vi "SetLaserConfigLCDC501.vi"(2 "LASER CONFIGURATION":T1={"LD Range"=1, "Laser Control Mode"=0, "Laser Mod On/OFF"=1, "Laser Mod BW"=1} {"Laser Mod BW" items=["Low", "High"]; "Laser Mod On/OFF" items=["OFF", "ON"]; "Laser Control Mode" items=["CC", "CP"]; "LD Range" items=["250mA", "500mA"]}, 8 "error in (no error)":errorcluster, 11 "VISA resource name":refnum<visa-resource-name>) -> (0 "error out":errorcluster, 3 "VISA resource name out":refnum<visa-resource-name>)   [LabVIEW 2021]
panel:
  # "LD Currernt Range"
  # "Laser Control Mode"
  # "Laser Mod On/OFF"
  # "Laser Mod BW"
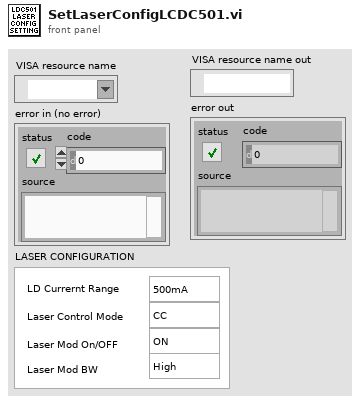
[diagram p1: front panel]
types:
  T1 = cluster{"LD Range":u16, "Laser Control Mode":u16, "Laser Mod On/OFF":u16, "Laser Mod BW":u16}
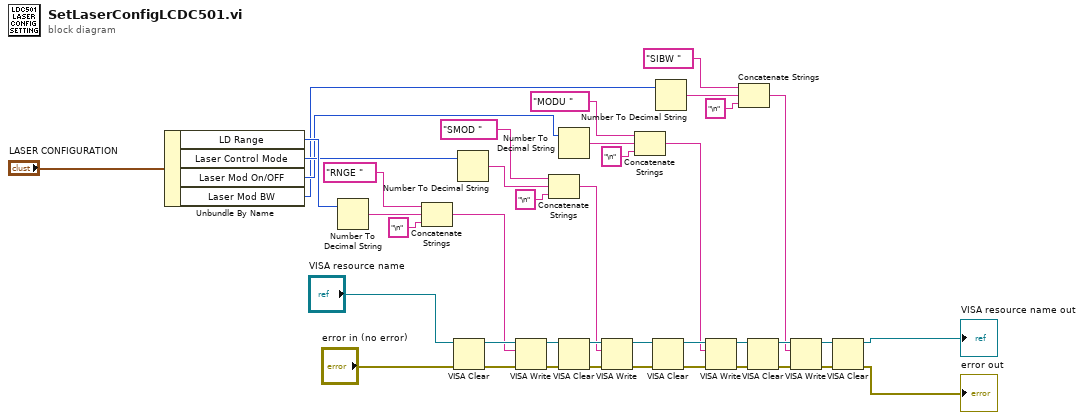
[diagram p0: block diagram]
diagram:
  n1 = Unbundle By Name("LASER CONFIGURATION") -> ("LD Range"=w6:u16, "Laser Control Mode"=w5:u16, "Laser Mod On/OFF"=w4:u16, "Laser Mod BW"=w3:u16)
  n2 = Number To Decimal String(number=w6) -> (decimal integer string=w31:string)  [unwired: 1 in]
  n3 = Concatenate Strings("RNGE " ("write buffer"), w31, "\n" ("string")) -> (w28:string)
  n4 = VISA Clear(VISA resource name="VISA resource name", error in (no error)="error in (no error)") -> (VISA resource name out=w40:refnum<visa-resource-name>, error out=w41:errorcluster)
  n5 = Number To Decimal String(number=w5) -> (decimal integer string=w26:string)  [unwired: 1 in]
  n6 = VISA Write(VISA resource name=w40, write buffer=w28, error in (no error)=w41) -> (VISA resource name out=w24:refnum<visa-resource-name>, error out=w23:errorcluster)  [unwired: 1 out]
  n7 = Concatenate Strings("SMOD " ("write buffer"), w26, "\n" ("string")) -> (w22:string)
  n8 = Number To Decimal String(number=w4) -> (decimal integer string=w17:string)  [unwired: 1 in]
  n9 = VISA Clear(VISA resource name=w24, error in (no error)=w23) -> (VISA resource name out=w38:refnum<visa-resource-name>, error out=w39:errorcluster)
  n10 = VISA Write(VISA resource name=w38, write buffer=w22, error in (no error)=w39) -> (VISA resource name out=w21:refnum<visa-resource-name>, error out=w20:errorcluster)  [unwired: 1 out]
  n11 = Concatenate Strings("MODU " ("write buffer"), w17, "\n" ("string")) -> (w16:string)
  n12 = VISA Clear(VISA resource name=w21, error in (no error)=w20) -> (VISA resource name out=w36:refnum<visa-resource-name>, error out=w37:errorcluster)
  n13 = Number To Decimal String(number=w3) -> (decimal integer string=w12:string)  [unwired: 1 in]
  n14 = VISA Write(VISA resource name=w36, write buffer=w16, error in (no error)=w37) -> (VISA resource name out=w15:refnum<visa-resource-name>, error out=w14:errorcluster)  [unwired: 1 out]
  n15 = Concatenate Strings("SIBW " ("write buffer"), w12, "\n" ("string")) -> (w10:string)
  n16 = VISA Clear(VISA resource name=w15, error in (no error)=w14) -> (VISA resource name out=w34:refnum<visa-resource-name>, error out=w35:errorcluster)
  n17 = VISA Write(VISA resource name=w34, write buffer=w10, error in (no error)=w35) -> (VISA resource name out=w9:refnum<visa-resource-name>, error out=w8:errorcluster)  [unwired: 1 out]
  n18 = VISA Clear(VISA resource name=w9, error in (no error)=w8) -> (VISA resource name out=→"VISA resource name out":refnum<visa-resource-name>, error out=→"error out":errorcluster)
